vi "ADS Get  Result.vi"(10 "ref in":u64, 11 "no_of_detections":i32) -> (2 "arry_cluster":T1(array[cluster]), 3 "ref out":u64)   [LabVIEW 2024]
uses:
  dependencies_dll_release/TCV_Lib.dll
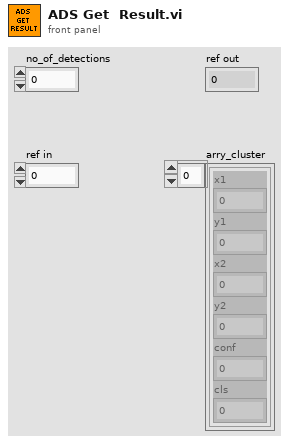
[diagram p1: front panel]
types:
  T1 = cluster{"x1":sgl, "y1":sgl, "x2":sgl, "y2":sgl, "conf":sgl, "cls":i32}[]
  T2 = cluster{"x1":sgl, "y1":sgl, "x2":sgl, "y2":sgl, "conf":sgl, "cls":i32}
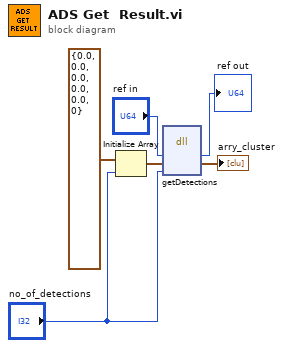
[diagram p0: block diagram]
diagram:
  n1 = Initialize Array(T2 {"x1"=0.0, "y1"=0.0, "x2"=0.0, "y2"=0.0, "conf"=0.0, "cls"=0}, "no_of_detections") -> (w2:T1)
  n2 = dll-call lib="D:/labviewTestTCVdll/TransformCV-LabVIEW/Test/dependencies_dll_release/TCV_Lib.dll" fn="getDetections"("ref"="ref in", "arry_cluster"=w2, "numberofdetection"="no_of_detections") -> ("ref"=→"ref out":u64, "arry_cluster"=→"arry_cluster":T1)  [unwired: 5 in, 2 out]
